vi "OLD Launch Wrapper.vi"(9 "Alias":string, 10 "Queue Actor":refnum<class "Queue Actor.lvclass">) -> ()   [LabVIEW 2021, in "jettl.lvlib" / "jettl Queue Actor.lvlib" / "jettl Queue Actor.lvclass"]
uses:
  jettl Queue Actor.lvclass
  Actor/Queue Actor/Queue Actor.lvclass
  C:/git/jettl/src/Actor/Actor/Actor.lvclass
  State/Teardown State/Teardown State.lvclass
  C:/git/jettl/src/jettl/jettl Queue Actor/State/State/State.lvclass
  jettl Queue Actor.lvclass/jettl Queue Actor.ctl
  jettl.lvlib
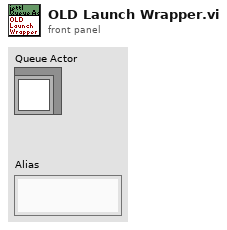
[diagram p1: front panel]
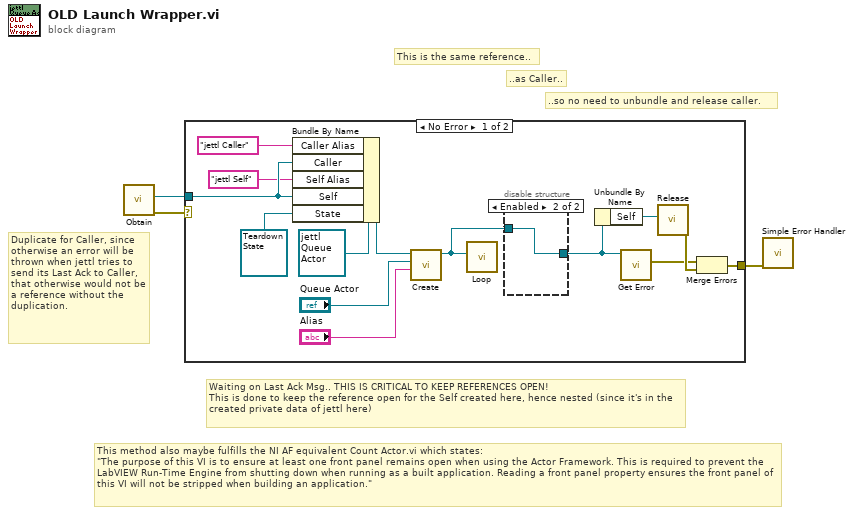
[diagram p0: block diagram]
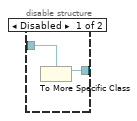
[diagram p2: hidden frame]
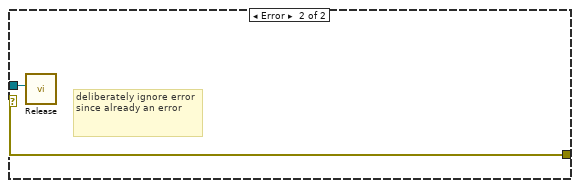
[diagram p3: hidden frame]
diagram:
  # "Duplicate for Caller, since otherwise an error will be thrown when jettl tries to send its Last Ack to Caller, that otherwise would not be a reference without the duplication."
  # "..so no need to unbundle and release caller."
  # "This is the same reference.."
  # "..as Caller.."
  # "Waiting on Last Ack Msg.. THIS IS CRITICAL TO KEEP REFERENCES OPEN!\nThis is done to keep the reference open for the Self created here, hence nested (since it's in the created private data of jettl here)"
  # "This method also maybe fulfills the NI AF equivalent Count Actor.vi which states:\n\"The purpose of this VI is to ensure at least one front panel remains open when using the Actor Framework. This is required to prevent the LabVIEW Run-Time Engine from shutting down when running as a built application. Reading a front panel property ensures the front panel of this VI will not be stripped when building an application.\""
  n1 = call "Obtain.vi"() -> ("error out"=w1:errorcluster, "Queue"=w3:refnum<data-value>)  [unwired: 10 in]
  n2 = case shown="No Error" w1 {
    selector: w1 -> [_ w21]
    tunnel: w3 -> [w7 w22]
    tunnel: [w16 w21] -> w2
    frame No Error {
      n3 = Bundle By Name(cluster=refnum<class "jettl Queue Actor.lvclass"> refnum ("Self Actor in"), "Caller Alias"="jettl Caller" ("Self Alias"), "Caller"=w7, "Self Alias"="jettl Self", "Self"=w7, "State"=refnum<class "Teardown State.lvclass"> refnum ("jettl.lvlib:Destroy State.lvclass")) -> (w15:refnum<class "jettl Queue Actor.lvclass">)
      n4 = call-dynamic "Create.vi"("Alias"="Alias", "Actor"="Queue Actor", "jettl Queue Actor in"=w15) -> ("jettl Queue Actor out"=w5:refnum<class "jettl Queue Actor.lvclass">)  [unwired: 8 in]
      n5 = call "Loop.vi"("Actor"=w5) -> ()  [unwired: 11 in]
      n6 = disable-structure shown="Enabled" {
        disable-tunnel: [w19 w20] -> w10
        disable-tunnel: w5 -> [w18 w20]
        frame Disabled {
          n7 = To More Specific Class(target class=w18) -> (specific class reference=w19:refnum<class "jettl Queue Actor.lvclass">)  [unwired: 2 in, 1 out]
        }
        frame Enabled {
        }
      }
      n8 = Unbundle By Name(w10) -> ("Self"=w17:refnum<data-value>)
      n9 = call-dynamic "Get Error.vi"("jettl Queue Actor in"=w10) -> ("Error"=w4:errorcluster)  [unwired: 10 in]
      n10 = call "Release.vi"("Queue"=w17) -> ("error out"=w11:errorcluster)  [unwired: 10 in]
      n11 = Merge Errors(w4, w11) -> (w16:errorcluster)
    }
    frame Error {
      # "deliberately ignore error since already an error"
      n12 = call "Release.vi"("Queue"=w22) -> ()  [unwired: 10 in, 1 out]
    }
  }
  n13 = call <vilib>:"Simple Error Handler.vi"("error in (no error)"=w2) -> ()  [unwired: 4 in, 5 out]
